vi "Request.vi"(8 "error in (no error)":errorcluster, 10 "request":refnum<class "request.lvclass">, 11 "output_actor in":refnum<class "test_hardwareactor.lvclass">) -> (0 "error out":errorcluster, 3 "output_actor out":refnum<class "test_hardwareactor.lvclass">)   [LabVIEW 2015, in "test_hardwareactor.lvclass"]
uses:
  test_hardwareactor.lvclass
  Request/request.lvclass
  Output Actor Hardware/Output Actor Hardware.lvclass
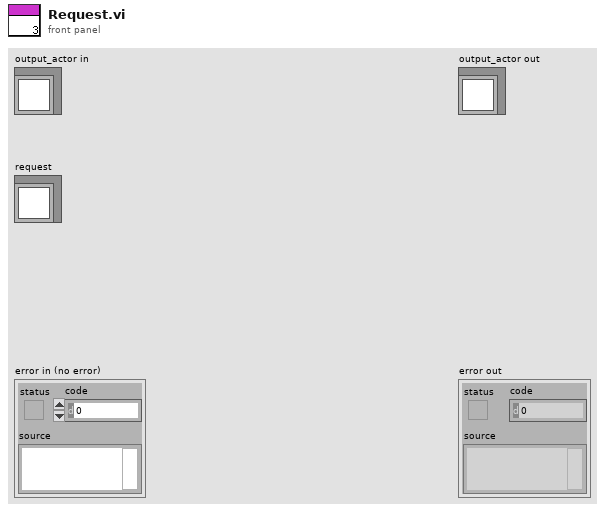
[diagram p1: front panel]
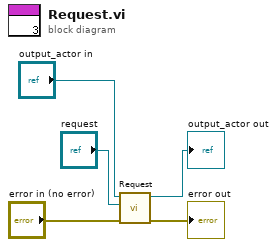
[diagram p0: block diagram]
diagram:
  n1 = call-parent "Request.vi"("error in (no error)"="error in (no error)", "request"="request", "output_actor in"="output_actor in") -> ("error out"=→"error out":errorcluster, "output_actor out"=→"output_actor out":refnum<class "test_hardwareactor.lvclass">)  [unwired: 7 in]
